vi "Washer HCC GUI.vi"(0 "Washer In":T1 {"Cycle Count" format="%05d"}, 2 "Enum":T5, 5 "Station Number In":string, 7 "New Washer Details In":T2, 9 "Com Port In":u8=13, 11 "Washer Status Serial Data In":T3, 12 "Agilent Data In":dbl[](array[numeric])=[1.0, 2.0, 3.0, 4.0, 5.0], 13 "Sample Buf Limit":i32=1000) -> (4 "Washer Out":T1 {"Cycle Count" format="%05d"}, 8 "New Dryer Testing File Init":bool, 10 "Restart Ready?":bool)   [LabVIEW 2009]
uses:
  Dryer Wilt/Update Wilt GUI Control.ctl
  Washer.ctl
  Dryer Wilt/Dryer Details.ctl
  Dryer Wilt/Dryer Com Port Info.ctl
  Dryer Wilt/Dryer Status Ctrl.ctl
  Globals HCC.vi
panel:
  out "Dryer Out.Sample Record(t, CC, Tc, ASCII, Status, L1,L2,Trmb,V{,V2,SW} ) 2":string[](array[string])
  out "Washer Out.Sample Record(t, CC, ASCII, Status )":string[](array[string])
  in  "Dryer Out":T1 {"Cycle Count" format="%05d"}
  in  "Tab Control":enum32{"Out", "In"}(tab)
  out "Washer Out  Breakout":T1 {"Cycle Count" format="%05d"}
  out "Washer In  Breakout":T6 {"Cycle Count" format="%05d"}
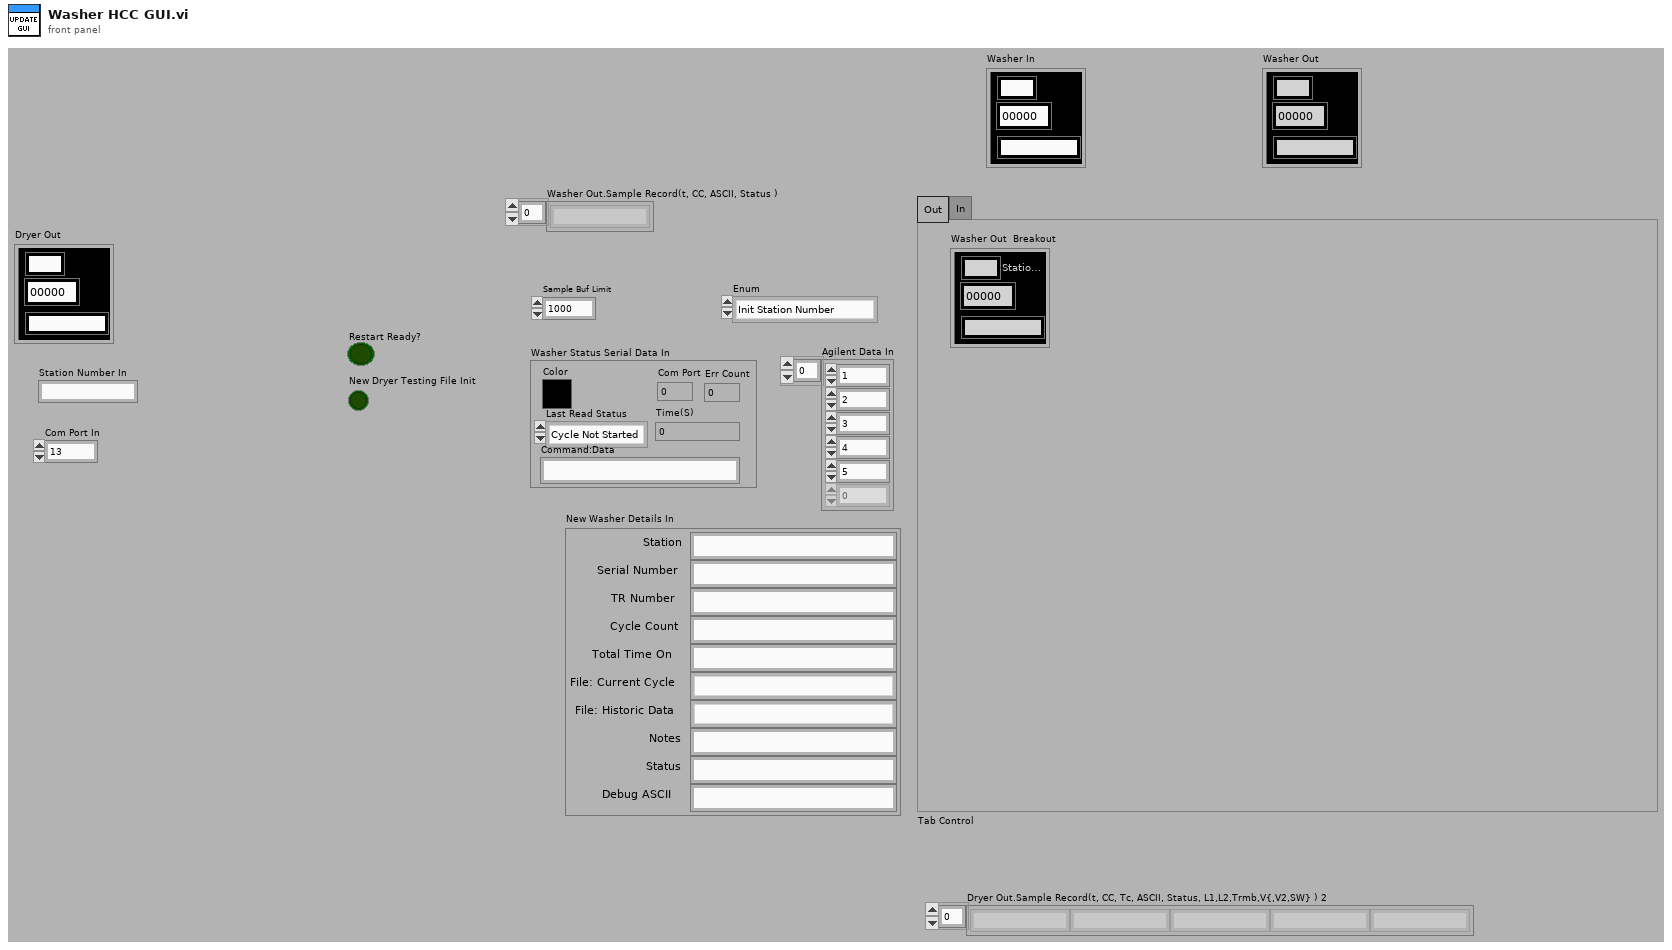
[diagram p1: front panel]
types:
  T1 = typedef "Washer.ctl" = cluster{"Serial Number":string, "Cycle Count":i32, "Station Number":string, "Dryer Details":T2, "Sample Record(t, CC, ASCII, Status ) ":string[], "Hist Record(Cycle Count, t-comp) ":string[][], "Status Color":u32, "Com Port":u8, "Bad Com Count":i32, "Boolean":bool}
  T2 = typedef "Dryer Details.ctl" = cluster{"Station":string, "Cycle Count":string, "Status":string, "Debug ASCII":string, "Notes":string, "File: Current Cycle":string, "Serial Number":string, "Total Time On":string, "TR Number":string, "File: Historic Data":string}
  T3 = typedef "Dryer Com Port Info.ctl" = cluster{"Color":u32, "Last Read Status":T4, "Command:Data":string, "Com Port":u8, "Time(S)":dbl, "Err Count":u8}
  T4 = typedef "Dryer Status Ctrl.ctl" = enum16{"Cycle Not Started", "Cycle Running", "Paused", "Cycle Completed", "Eval Mode Entered", "Err"}
  T5 = typedef "Update Wilt GUI Control.ctl" = enum16{"Init Station Number", "Update Detail Data", "Update Status", "Init Com Port Num", "Update Sample Info"}
  T6 = cluster{"Serial Number":string, "Cycle Count":i32, "Station Number":string, "Dryer Details":T2, "Sample Record(t, CC, Tc, ASCII, Status, L1,L2,Trmb,V{,V2,SW} ) ":string[], "Hist Record(Cycle Count, t-comp,L1max, L2max, Tmax) ":string[][], "Status Color":u32, "Com Port":u8, "Bad Com Count":i32, "Boolean":bool}
  T7 = cluster{"New Washer Details In":T2, "Station Number In":string, "Com Port In":u8, "Agilent Data In":dbl[], "Washer Status Serial Data In":T3, "Restart Ready?":bool, "Dryer Out":T1, "Sample Buf Limit":i32, "Temperature Fault":bool}
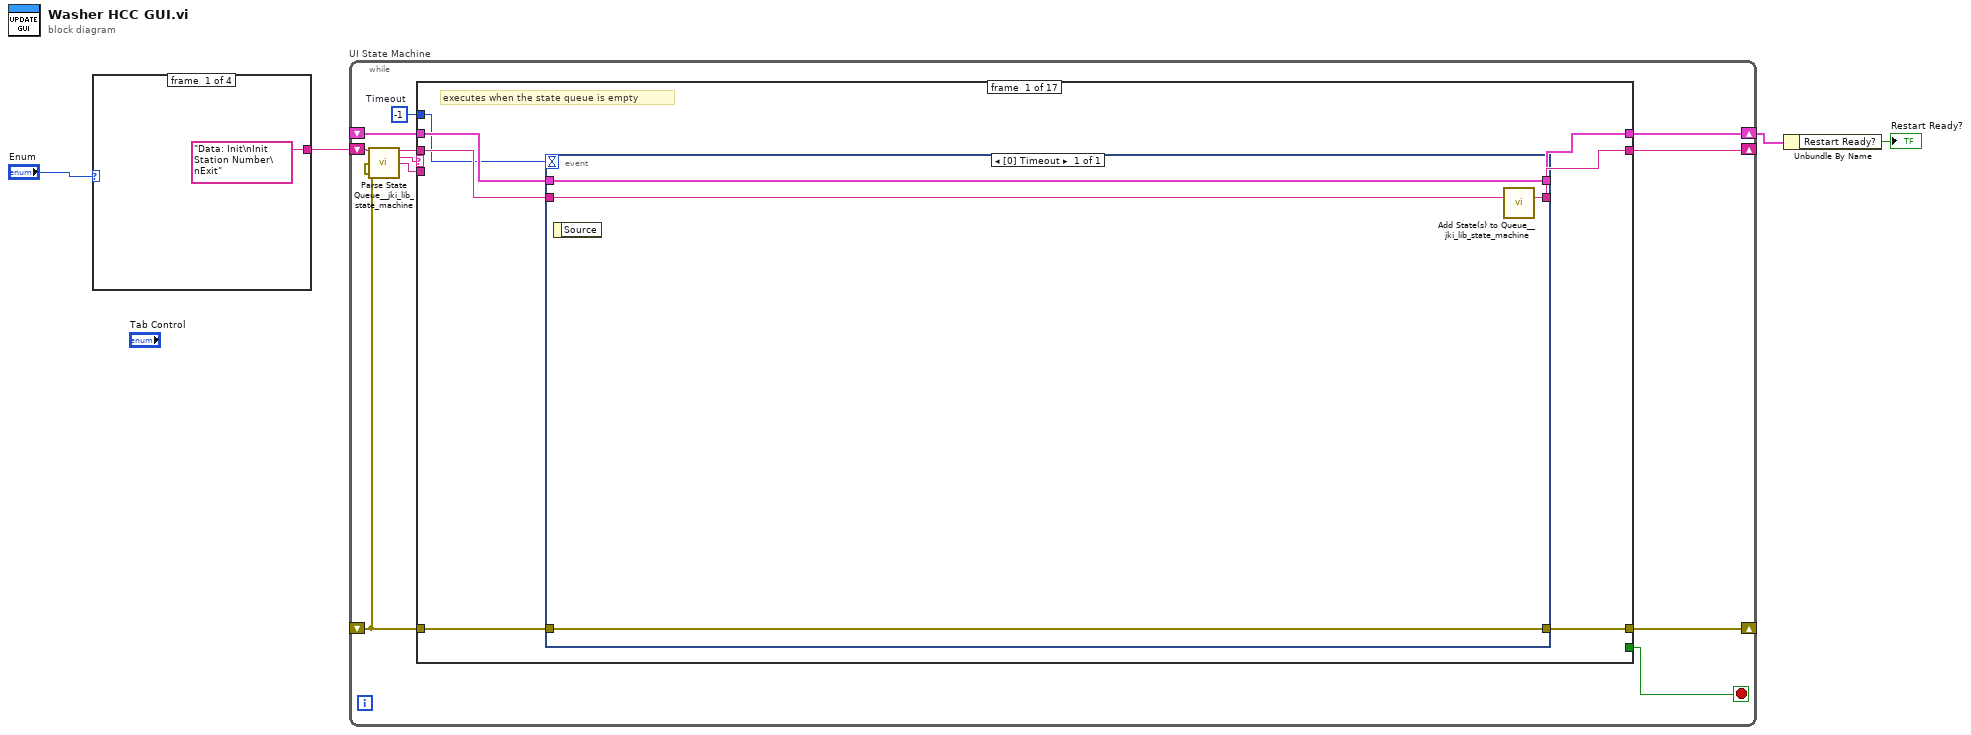
[diagram p0: block diagram]
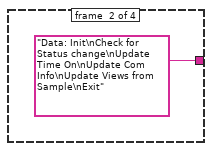
[diagram p2: hidden frame]
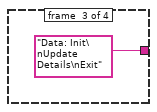
[diagram p3: hidden frame]
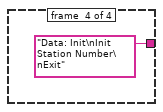
[diagram p4: hidden frame]
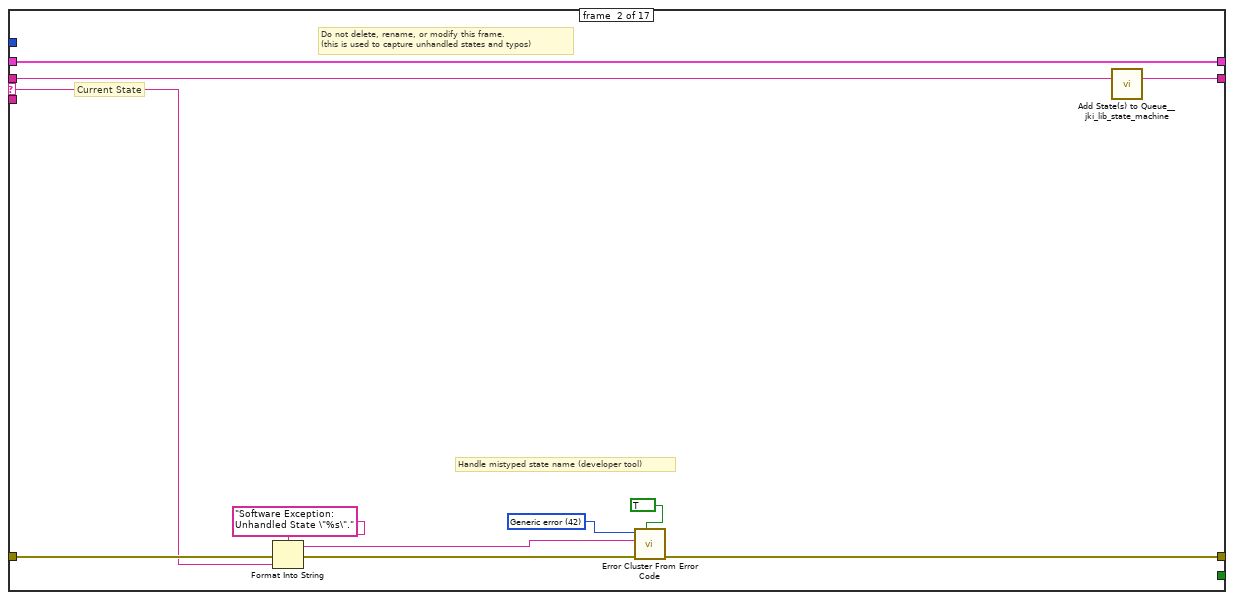
[diagram p5: hidden frame]
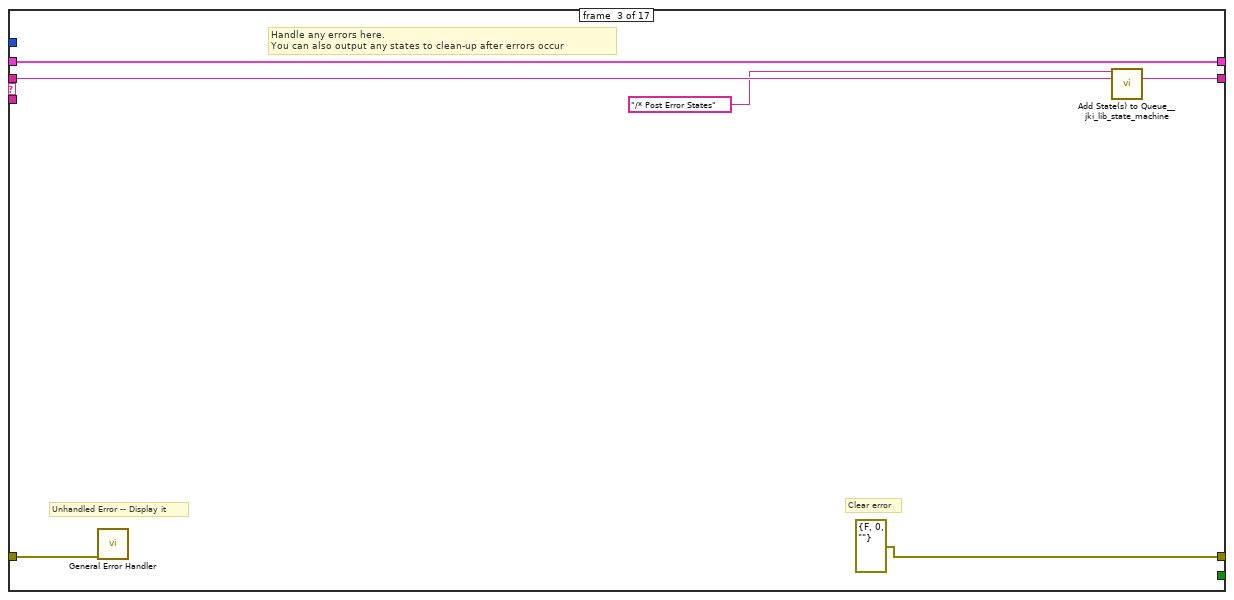
[diagram p6: hidden frame]
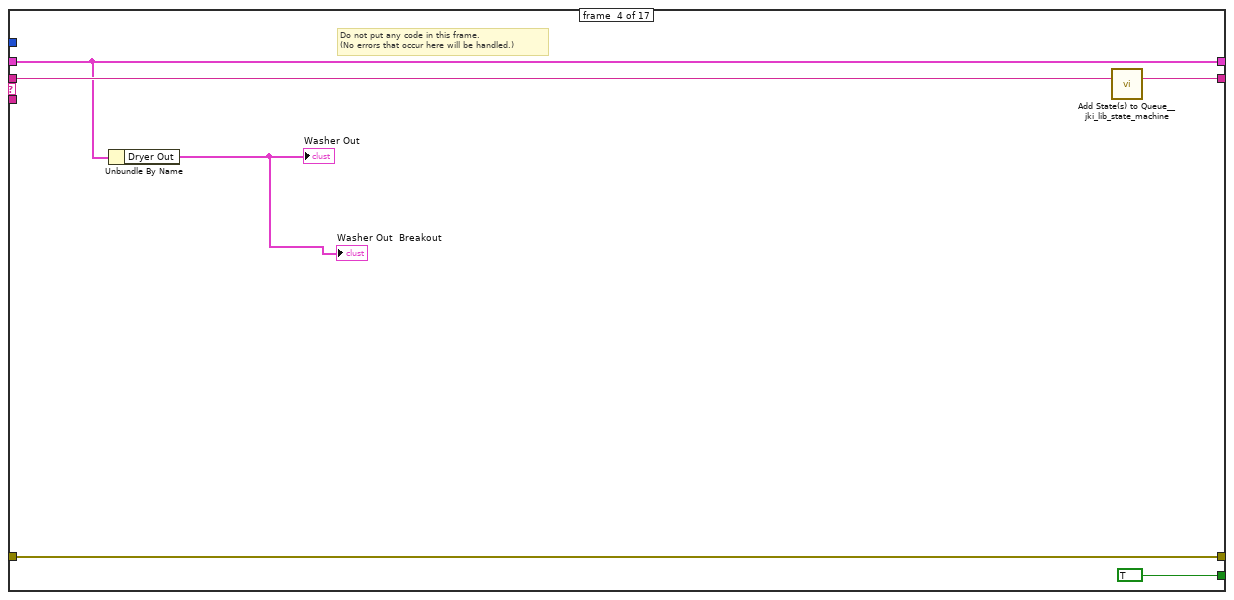
[diagram p7: hidden frame]
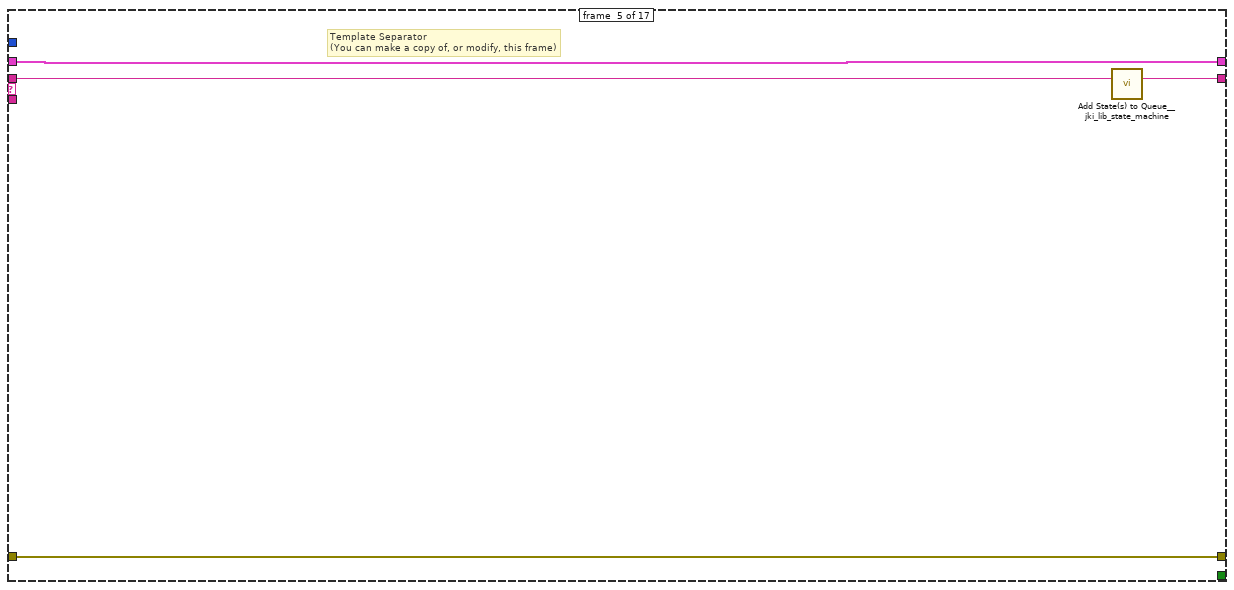
[diagram p8: hidden frame]
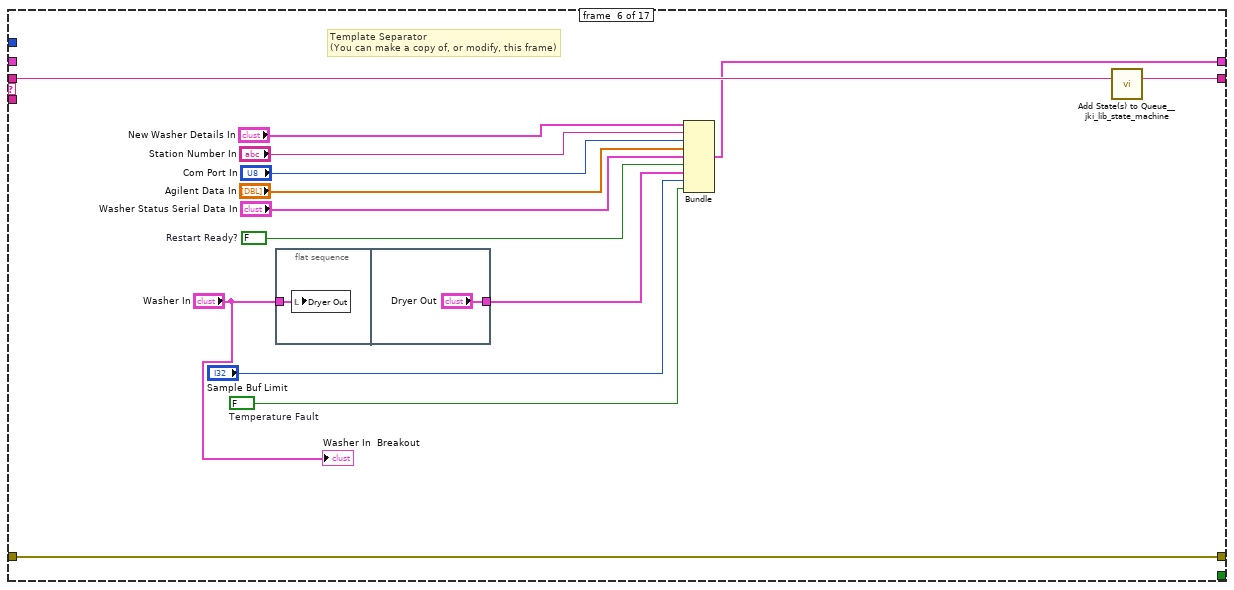
[diagram p9: hidden frame]
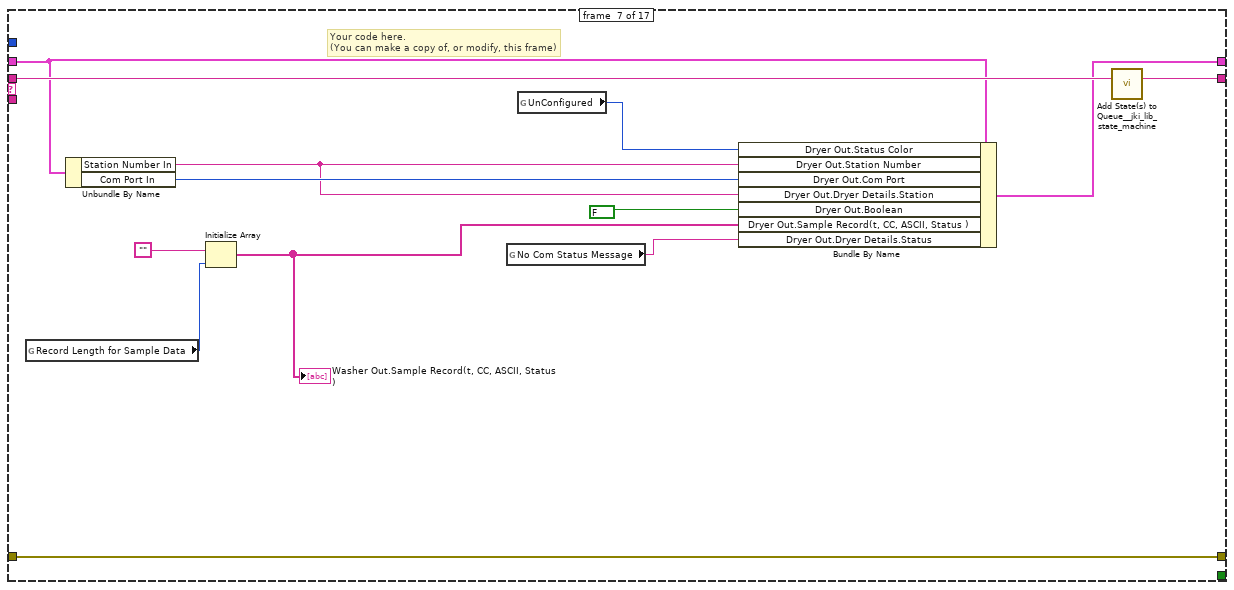
[diagram p10: hidden frame]
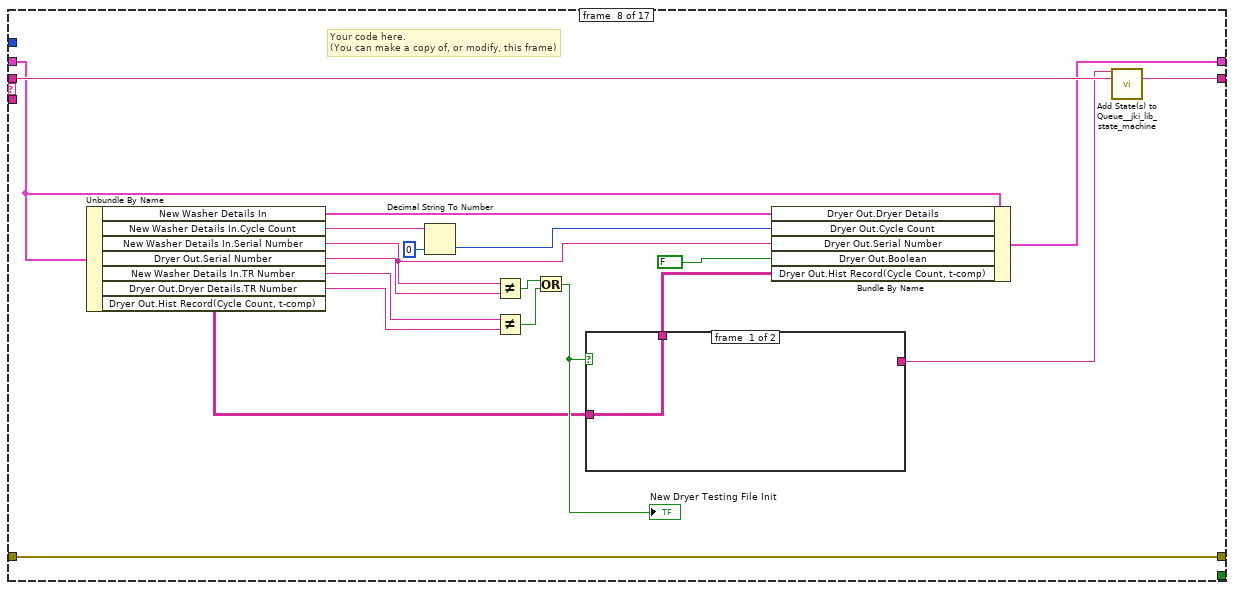
[diagram p11: hidden frame]
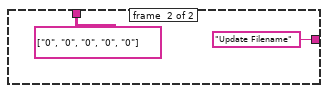
[diagram p12: hidden frame]
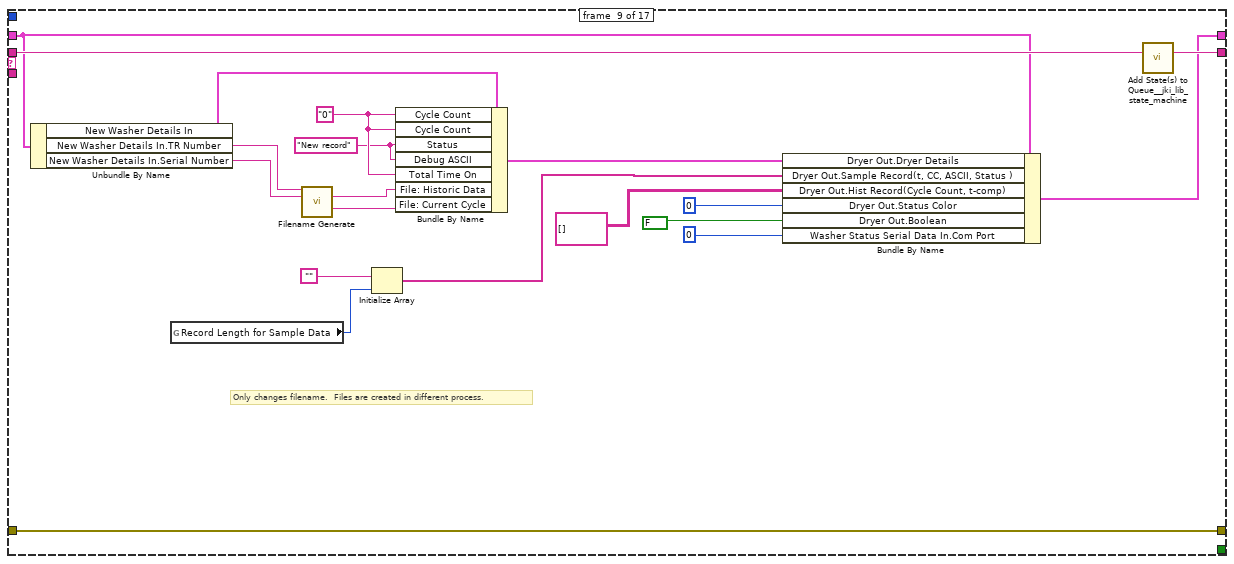
[diagram p13: hidden frame]
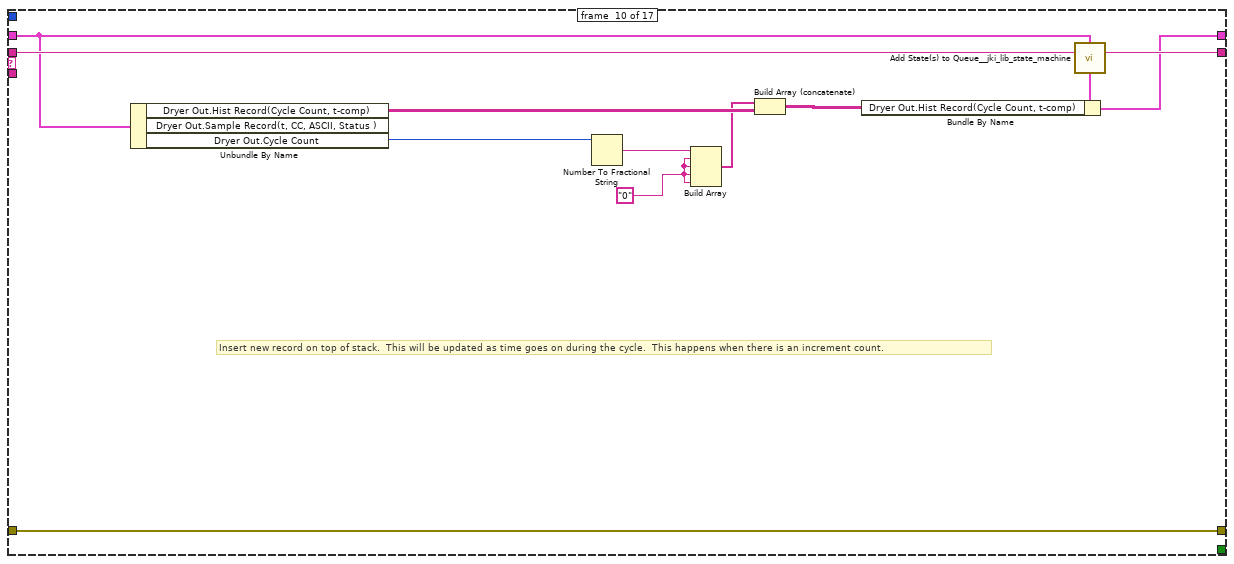
[diagram p14: hidden frame]
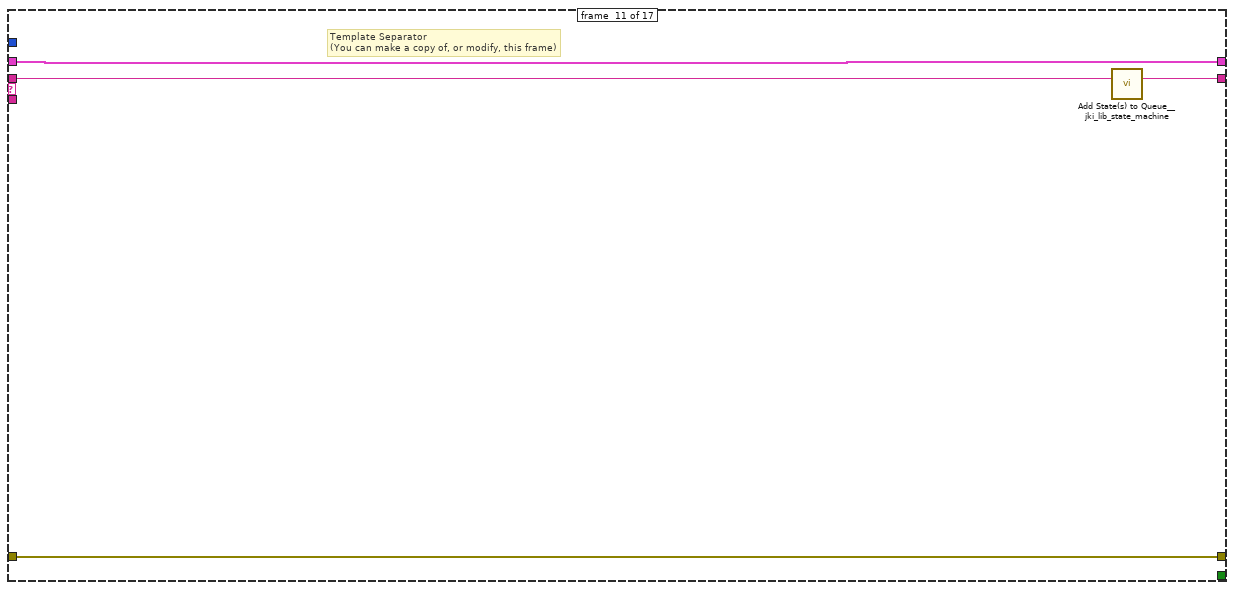
[diagram p15: hidden frame]
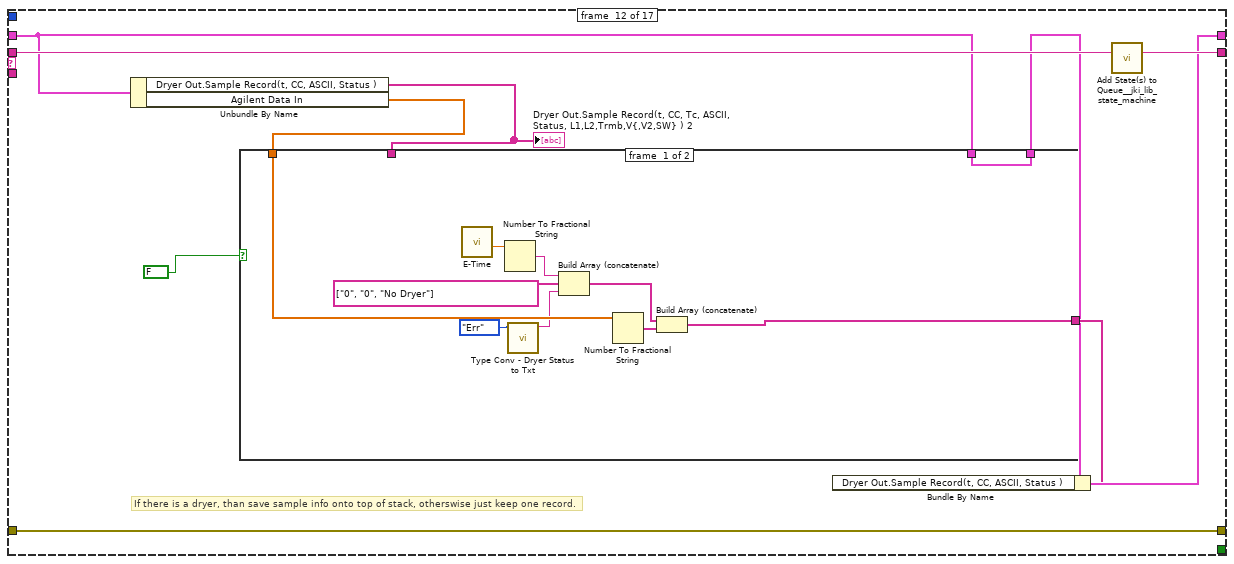
[diagram p16: hidden frame]
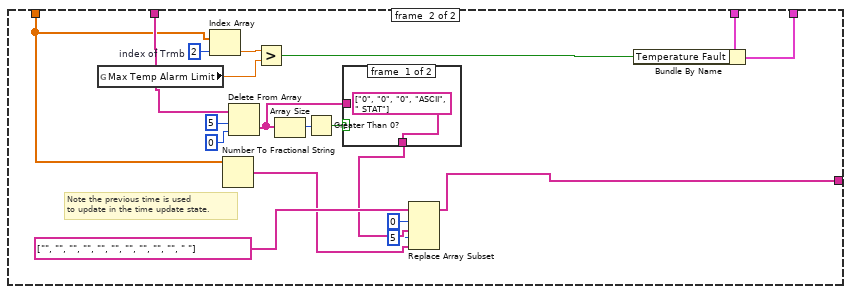
[diagram p17: hidden frame]
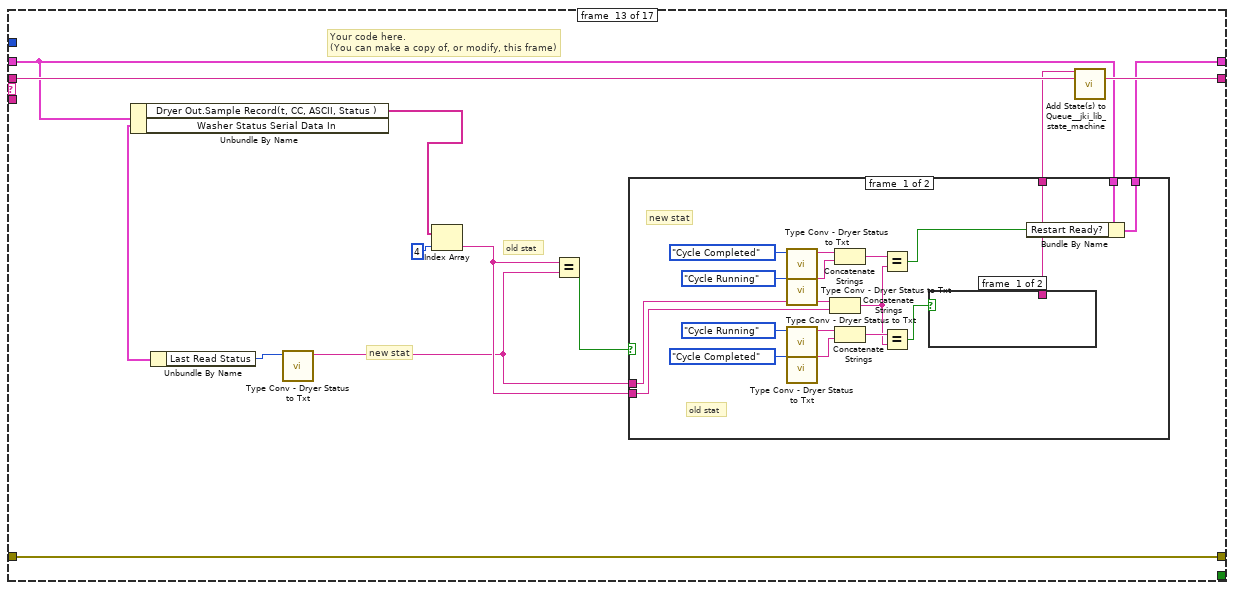
[diagram p19: hidden frame]
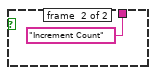
[diagram p20: hidden frame]
diagram:
  n1 = case shown="\"Update Detail Data\"" "Enum" {
    tunnel: ["Data: Init\nInit Station Number\nExit" ("States Out") "Data: Init\nCheck for Status change\nUpdate Time On\nUpdate Com Info\nUpdate Views from Sample\nExit" ("States Out") "Data: Init\nUpdate Details\nExit" ("States Out") "Data: Init\nInit Station Number\nExit" ("States Out")] -> w3
    frame #0 {
    }
    frame #1 {
    }
    frame #2 {
    }
    frame #3 {
    }
  }
  n2 = while "UI State Machine" {
    shift-right: [w12] -> w2
    shift-left: _ -> [w11]
    shift-right: [w15] -> _
    shift-left: _ -> [w9]
    shift-right: [w14] -> _
    shift-left: w3 -> [w16]
    stop <- w13 stop-if-true
    w10 = -1  # Timeout
    n3 = call <vilib>:"Parse State Queue__jki_lib_state_machine.vi"("State Queue"=w16, "Error In (no error)"=w9) -> ("Remaining States"=w18:string, "Current State"=w19:string, "Arguments"=w17:string)  [unwired: 11 in]
    n4 = case shown="\"Update Details\"" w19 {
      selector: w19 -> [_ w31 _ _ _ _ _ _ _ _ _ _ _ _ _ _ _]
      tunnel: w18 -> [w26 w35 w47 w53 w57 w71 w86 w106 w129 w140 w144 w154 w198 w229 w273 w329 w341]
      tunnel: w17 -> [_ _ _ _ _ _ _ _ _ _ _ _ _ _ _ _ _]
      tunnel: w11 -> [w24 w33 w44 w49 w54 _ w83 w97 w126 w137 w141 w146 w190 w222 w270 w326 w337]
      tunnel: [w23 w37 errorcluster {"status"=FALSE, "code"=0, "source"=""} ("error out") w51 w55 w69 w84 w104 w127 w138 w142 w152 w196 w227 w271 w327 w339] -> w15
      tunnel: w9 -> [w22 w36 w43 w51 w55 w69 w84 w104 w127 w138 w142 w152 w196 w227 w271 w327 w339]
      tunnel: [w25 w34 w46 w52 w56 w70 w85 w105 w128 w139 w143 w153 w197 w228 w272 w328 w340] -> w14
      tunnel: [_ _ _ TRUE _ _ _ _ _ _ _ _ _ _ _ _ _] -> w13
      tunnel: [w21 w33 w44 w49 w54 w68 w82 w103 w125 w136 w141 w151 w189 w221 w269 w325 w336] -> w12
      tunnel: w10 -> [w20 _ _ _ _ _ _ _ _ _ _ _ _ _ _ _ _]
      frame #0 {
        # "executes when the state queue is empty"
        n5 = event shown="[0] Timeout" {
          selector: _ -> [_]
          dyn-events: _ -> [_]
          timeout: w20 -> [_]
          tunnel: w26 -> [w30]
          tunnel: [w29] -> w25
          tunnel: w24 -> [w27]
          tunnel: [w28] -> w23
          tunnel: w22 -> [w28]
          tunnel: [w27] -> w21
          event [0] Timeout {
            n6 = event-data() -> ()  [unwired: 1 in, 1 out]
            n7 = call <vilib>:"Add State(s) to Queue__jki_lib_state_machine.vi"("State(s) in (\"\")"=w30) -> ("States Out"=w29:string)  [unwired: 14 in]
          }
        }
      }
      frame #1 {
        w40 = 42 items=["No error", "Argument error", "Memory is full", "Out of zone", "End of file", "File already open", "Generic file I/O error", "File not found", "File permission error", "Disk is full", "Duplicate path", "Too many files open", "System feature not enabled", "Resource file not found", "Cannot add resource", "Resource not found", "Image not found", "Image memory error", "Pen does not exist", "Config type invalid", "Config token not found", "Config parse error", "Config memory error", "Bad external code format", "Bad external code offset", "External code not present", "Null window", "Destroy window error", "Null menu", "Print aborted", "Bad print record", "Print driver error", "Windows error during printing", "Memory error during printing", "Print dialog error", "Generic print error", "Invalid device refnum", "Device not found", "Device parameter error", "Device unit error", "Cannot open device", "Device call aborted", "Generic error", "Cancelled by user", "Object ID too low", "Object ID too high", "Object not in heap", "Unknown heap", "Unknown object (invalid DefProc)", "Unknown object (DefProc not in table)", "Message out of range", "Invalid (null) method", "Unknown message", "Manager call not supported", "Bad address", "Network operation in progress", "Network operation timed out", "Connection is busy", "Network attribute not supported", "Network error", "Address in use", "System out of memory", "Connection aborted", "Connection refused", "Not connected", "Already connected", "Connection closed", "Initialization error (interapplication manager)", "Bad occurrence", "Wait on unbound occurrence handler", "Occurrence queue overflow", "Datalog type conflict", "Unused", "Unrecognized type (interapplication manager)", "Memory corrupt", "Failed to make temporary DLL", "Old CIN version", "Drag socket not found", "Failed to load drop-object", "Failed to register OLE object", "Failed to release OLE object", "Format specifier type mismatch", "Unknown format specifier", "Too few format specifiers", "Too many format specifiers", "Scan failed", "Newer CIN version", "Error converting to variant", "Runtime menu error", "Password tampered", "Variant attribute not found", "Incompatible variant data type", "Event data is not available", "Event Store is not present", "Occurrence is not found", "Event Queue is not created", "Event info is not available", "Refnum passed is NULL", "Error retrieving Class GUID", "Error retrieving CoClass GUID", "Error retrieving TypeLib GUID.", "Bad built application magic bytes.", "Specific driver is different from the specific driver associated with the Logical Name.", "There is no session opened to the class driver.", "Max Error", "MAX - Error with config objects", "MAX - Error loading configuration", "MAX - Group not supported"]
        # "Current State"
        # "Do not delete, rename, or modify this frame.\n(this is used to capture unhandled states and typos)"
        # "Handle mistyped state name (developer tool)"
        n8 = Format Into String(format string="Software Exception: Unhandled State \"%s\"." ("message"), error in=w36, w31) -> (resulting string=w39:string, error out=w38:errorcluster)  [unwired: 1 in]
        n9 = call <vilib>:"Error Cluster From Error Code.vi"("show call chain? (False)"=TRUE, "error in (no error)"=w38, "error message (\"\")"=w39, "error code (0)"=w40) -> ("error out"=w37:errorcluster)  [unwired: 5 in]
        n10 = call <vilib>:"Add State(s) to Queue__jki_lib_state_machine.vi"("State(s) in (\"\")"=w35) -> ("States Out"=w34:string)  [unwired: 14 in]
      }
      frame #2 {
        # "Unhandled Error -- Display it"
        # "Handle any errors here.\nYou can also output any states to clean-up after errors occur"
        # "Clear error"
        n11 = call <vilib>:"General Error Handler.vi"("error in (no error)"=w43) -> ()  [unwired: 10 in, 5 out]
        n12 = call <vilib>:"Add State(s) to Queue__jki_lib_state_machine.vi"("State(s) in Front (\"\")"="/* Post Error States", "State(s) in (\"\")"=w47) -> ("States Out"=w46:string)  [unwired: 13 in]
      }
      frame #3 {
        # "Do not put any code in this frame.\n(No errors that occur here will be handled.)"
        n13 = Unbundle By Name(w49) -> ("Dryer Out"=→"Washer Out" →"Washer Out  Breakout":T1)
        n14 = call <vilib>:"Add State(s) to Queue__jki_lib_state_machine.vi"("State(s) in (\"\")"=w53) -> ("States Out"=w52:string)  [unwired: 14 in]
      }
      frame #4 {
        # "Template Separator\n(You can make a copy of, or modify, this frame)"
        n15 = call <vilib>:"Add State(s) to Queue__jki_lib_state_machine.vi"("State(s) in (\"\")"=w57) -> ("States Out"=w56:string)  [unwired: 14 in]
      }
      frame #5 {
        w58 = FALSE  # Temperature Fault
        w62 = FALSE  # Restart Ready?
        # "Template Separator\n(You can make a copy of, or modify, this frame)"
        n16 = flat-sequence {
          tunnel: "Washer In" -> [w72]
          tunnel: ["Dryer Out"] -> w60
          frame #0 {
            n17 = local write "Dryer Out"(w72) -> ()
          }
          frame #1 {
          }
        }
        n18 = Bundle("New Washer Details In"="New Washer Details In", "Station Number In"="Station Number In", "Com Port In"="Com Port In", "Agilent Data In"="Agilent Data In", "Washer Status Serial Data In"="Washer Status Serial Data In", "Restart Ready?"=w62, "Dryer Out"=w60, "Sample Buf Limit"="Sample Buf Limit", "Temperature Fault"=w58) -> (w68:T7)  [unwired: 1 in]
        n19 = call <vilib>:"Add State(s) to Queue__jki_lib_state_machine.vi"("State(s) in (\"\")"=w71) -> ("States Out"=w70:string)  [unwired: 14 in]
        "Washer In  Breakout" <- "Washer In"
      }
      frame #6 {
        # "Your code here.\n(You can make a copy of, or modify, this frame)"
        n20 = global read "Globals HCC.vi" "Record Length for Sample Data"() -> (w75:i32)
        n21 = Unbundle By Name(w83) -> ("Station Number In"=w74:string, "Com Port In"=w81:u8)
        n22 = Initialize Array("", w75) -> (w76:string[])
        "Washer Out.Sample Record(t, CC, ASCII, Status )" <- w76
        n23 = global read "Globals HCC.vi" "No Com Status Message"() -> (w78:string)
        n24 = global read "Globals HCC.vi" "UnConfigured"() -> (w79:u32)
        n25 = Bundle By Name(cluster=w83, "Dryer Out.Status Color"=w79, "Dryer Out.Station Number"=w74, "Dryer Out.Com Port"=w81, "Dryer Out.Dryer Details.Station"=w74, "Dryer Out.Boolean"=FALSE ("Dryer In.Boolean"), "Dryer Out.Sample Record(t, CC, ASCII, Status )"=w76, "Dryer Out.Dryer Details.Status"=w78) -> (w82:T7)
        n26 = call <vilib>:"Add State(s) to Queue__jki_lib_state_machine.vi"("State(s) in (\"\")"=w86) -> ("States Out"=w85:string)  [unwired: 14 in]
      }
      frame #7 {
        # "Your code here.\n(You can make a copy of, or modify, this frame)"
        n27 = Unbundle By Name(w97) -> ("New Washer Details In"=w96:T2, "New Washer Details In.Cycle Count"=w93:string, "New Washer Details In.Serial Number"=w92:string, "Dryer Out.Serial Number"=w91:string, "New Washer Details In.TR Number"=w95:string, "Dryer Out.Dryer Details.TR Number"=w94:string, "Dryer Out.Hist Record(Cycle Count, t-comp)"=w87:string[][])
        n28 = Decimal String To Number(string=w93, default (0L)=0 ("default (0 I32)")) -> (number=w100:i32)  [unwired: 1 in, 1 out]
        n29 = Not Equal?(x=w92, y=w91) -> (x != y?=w90:bool)
        n30 = Not Equal?(x=w95, y=w94) -> (x != y?=w89:bool)
        n31 = Or(x=w90, y=w89) -> (x .or. y?=w101:bool)
        "New Dryer Testing File Init" <- w101
        n32 = case shown="False" w101 {
          tunnel: [_ "Update Filename"] -> w102
          tunnel: [w107 string[][] [["0", "0", "0", "0", "0"]] ("Hist Record(Cycle Count, t-comp,L1max, L2max, Tmax)")] -> w88
          tunnel: w87 -> [w107 _]
          frame #0 {
          }
          frame #1 {
          }
        }
        n33 = Bundle By Name(cluster=w97, "Dryer Out.Dryer Details"=w96, "Dryer Out.Cycle Count"=w100, "Dryer Out.Serial Number"=w92, "Dryer Out.Boolean"=FALSE ("Dryer In.Boolean"), "Dryer Out.Hist Record(Cycle Count, t-comp)"=w88) -> (w103:T7)
        n34 = call <vilib>:"Add State(s) to Queue__jki_lib_state_machine.vi"("State(s) in Front (\"\")"=w102, "State(s) in (\"\")"=w106) -> ("States Out"=w105:string)  [unwired: 13 in]
      }
      frame #8 {
        w123 = "New record" ("Status")
        w124 = "0" ("Cycle Count")
        # "Only changes filename.  Files are created in different process."
        n35 = Unbundle By Name(w126) -> ("New Washer Details In"=w121:T2, "New Washer Details In.TR Number"=w119:string, "New Washer Details In.Serial Number"=w118:string)
        n36 = global read "Globals HCC.vi" "Record Length for Sample Data"() -> (w110:i32)
        n37 = call "Filename Generate.vi"("TR Number"=w119, "Serial Number"=w118) -> ("Filename for Hist data"=w120:string, "Filename for Samples"=w113:string)  [unwired: 10 in, 2 out]
        n38 = Initialize Array("", w110) -> (w111:string[])
        n39 = Bundle By Name(cluster=w121, "Cycle Count"=w124, "Cycle Count"=w124, "Status"=w123, "Debug ASCII"=w123, "Total Time On"=w124, "File: Historic Data"=w120, "File: Current Cycle"=w113) -> (w122:T2)
        n40 = Bundle By Name(cluster=w126, "Dryer Out.Dryer Details"=w122, "Dryer Out.Sample Record(t, CC, ASCII, Status )"=w111, "Dryer Out.Hist Record(Cycle Count, t-comp)"=string[][] [] ("Dryer In.Sample Record(t, CC, Tc, ASCII, Status, L1,L2,Trmb,V{,V2,SW} )"), "Dryer Out.Status Color"=u32 0 ("Dryer In.Status Color"), "Dryer Out.Boolean"=FALSE ("Dryer In.Boolean"), "Washer Status Serial Data In.Com Port"=u8 0 ("Dryer In.Com Port")) -> (w125:T7)
        n41 = call <vilib>:"Add State(s) to Queue__jki_lib_state_machine.vi"("State(s) in (\"\")"=w129) -> ("States Out"=w128:string)  [unwired: 14 in]
      }
      frame #9 {
        w130 = "0" ("element")
        # "Insert new record on top of stack.  This will be updated as time goes on during the cycle.  This happens when there is an increment count."
        n42 = Unbundle By Name(w137) -> ("Dryer Out.Hist Record(Cycle Count, t-comp)"=w134:string[][], "Dryer Out.Cycle Count"=w131:i32)  [unwired: 1 out]
        n43 = Number To Fractional String(number=w131) -> (F-format string=w135:string)  [unwired: 3 in]
        n44 = Build Array(w135, w130, w130, w130, w130) -> (w133:string[])
        n45 = Build Array (concatenate)(w133, w134) -> (w132:string[][])
        n46 = Bundle By Name(cluster=w137, "Dryer Out.Hist Record(Cycle Count, t-comp)"=w132) -> (w136:T7)
        n47 = call <vilib>:"Add State(s) to Queue__jki_lib_state_machine.vi"("State(s) in (\"\")"=w140) -> ("States Out"=w139:string)  [unwired: 14 in]
      }
      frame #10 {
        # "Template Separator\n(You can make a copy of, or modify, this frame)"
        n48 = call <vilib>:"Add State(s) to Queue__jki_lib_state_machine.vi"("State(s) in (\"\")"=w144) -> ("States Out"=w143:string)  [unwired: 14 in]
      }
      frame #11 {
        # "If there is a dryer, than save sample info onto top of stack, otherswise just keep one record."
        n49 = Unbundle By Name(w146) -> ("Dryer Out.Sample Record(t, CC, ASCII, Status )"=w148:string[], "Agilent Data In"=w150:dbl[])
        "Dryer Out.Sample Record(t, CC, Tc, ASCII, Status, L1,L2,Trmb,V{,V2,SW} ) 2" <- w148
        n50 = case shown="False" FALSE {
          tunnel: w150 -> [w164 w171]
          tunnel: [w156 w172] -> w149
          tunnel: w148 -> [_ w173]
          tunnel: w146 -> [w155 w167]
          tunnel: [w155 w166] -> w145
          frame #0 {
            n51 = call "E-Time.vi"() -> ("Elapsed Time (sec)"=w158:dbl)  [unwired: 9 in, 2 out]
            n52 = Number To Fractional String(number=w158) -> (F-format string=w157:string)  [unwired: 3 in]
            n53 = call "Type Conv - Dryer Status to Txt.vi"("Status"=Dryer_Status_Ctrl."Err") -> ("Ring Text.Text"=w160:string)  [unwired: 10 in]
            n54 = Build Array (concatenate)(w157, string[] ["0", "0", "No Dryer"], w160) -> (w159:string[])
            n55 = Number To Fractional String(number=w164) -> (F-format string=w163:string[])  [unwired: 3 in]
            n56 = Build Array (concatenate)(w159, w163) -> (w156:string[])
          }
          frame #1 {
            w170 = 2  # index of Trmb
            # "Note the previous time is used\nto update in the time update state."
            n57 = global read "Globals HCC.vi" "Max Temp Alarm Limit"() -> (w168:dbl)
            n58 = Index Array(array=w171, index=w170) -> (element=w169:dbl)
            n59 = Number To Fractional String(number=w171) -> (F-format string=w174:string[])  [unwired: 3 in]
            n60 = Delete From Array(array=w173, length=5, index=0) -> (deleted portion=w179:string[])  [unwired: 1 out]
            n61 = Greater?(x=w169, y=w168) -> (0:w165:bool)
            n62 = Array Size(array=w179) -> (size(s)=w181:i32)
            n63 = Greater Than 0?(x=w181) -> (x > 0?=w180:bool)
            n64 = case shown="True" w180 {
              tunnel: [string[] ["0", "0", "0", "ASCII", " STAT"] w185] -> w176
              tunnel: w179 -> [_ w185]
              frame #0 {
              }
              frame #1 {
              }
            }
            n65 = Replace Array Subset(array=string[] ["", "", "", "", "", "", "", "", "", "", " "], new element #1=w176, index #1=0 ("index"), new element #2=w174, index #2=5 ("index")) -> (w172:string[])
            n66 = Bundle By Name(cluster=w167, "Temperature Fault"=w165) -> (w166:T7)
          }
        }
        n67 = Bundle By Name(cluster=w145, "Dryer Out.Sample Record(t, CC, ASCII, Status )"=w149) -> (w151:T7)
        n68 = call <vilib>:"Add State(s) to Queue__jki_lib_state_machine.vi"("State(s) in (\"\")"=w154) -> ("States Out"=w153:string)  [unwired: 14 in]
      }
      frame #12 {
        # "new stat"
        # "old stat"
        # "Your code here.\n(You can make a copy of, or modify, this frame)"
        n69 = Unbundle By Name(w190) -> ("Dryer Out.Sample Record(t, CC, ASCII, Status )"=w194:string[], "Washer Status Serial Data In"=w195:T3)
        n70 = Unbundle By Name(w195) -> ("Last Read Status"=w193:T4)
        n71 = call "Type Conv - Dryer Status to Txt.vi"("Status"=w193) -> ("Ring Text.Text"=w187:string)  [unwired: 10 in]
        n72 = Index Array(array=w194, index=4 ("disabled index (col)")) -> (element=w188:string)
        n73 = Equal?(x=w188, y=w187) -> (x = y?=w192:bool)
        n74 = case shown="False" w192 {
          tunnel: [w205 "" ("State(s) in Front (\"\")")] -> w191
          tunnel: w187 -> [w212 _]
          tunnel: w188 -> [w211 _]
          tunnel: w190 -> [w201 w218]
          tunnel: [w200 w218] -> w189
          frame #0 {
            # "new stat"
            # "old stat"
            n75 = call "Type Conv - Dryer Status to Txt.vi"("Status"=Dryer_Status_Ctrl."Cycle Completed") -> ("Ring Text.Text"=w209:string)  [unwired: 10 in]
            n76 = call "Type Conv - Dryer Status to Txt.vi"("Status"=Dryer_Status_Ctrl."Cycle Running") -> ("Ring Text.Text"=w210:string)  [unwired: 10 in]
            n77 = call "Type Conv - Dryer Status to Txt.vi"("Status"=Dryer_Status_Ctrl."Cycle Running") -> ("Ring Text.Text"=w214:string)  [unwired: 10 in]
            n78 = call "Type Conv - Dryer Status to Txt.vi"("Status"=Dryer_Status_Ctrl."Cycle Completed") -> ("Ring Text.Text"=w213:string)  [unwired: 10 in]
            n79 = Concatenate Strings(w212, w211) -> (w203:string)
            n80 = Concatenate Strings(w209, w210) -> (w206:string)
            n81 = Concatenate Strings(w214, w213) -> (w204:string)
            n82 = Equal?(x=w206, y=w203) -> (x = y?=w199:bool)
            n83 = Equal?(x=w204, y=w203) -> (x = y?=w202:bool)
            n84 = case shown="True" w202 {
              tunnel: [_ "Increment Count" ("State(s) in Front (\"\")")] -> w205
              frame #0 {
              }
              frame #1 {
              }
            }
            n85 = Bundle By Name(cluster=w201, "Restart Ready?"=w199) -> (w200:T7)
          }
          frame #1 {
            # "If status is the same,\ndon't do extra steps."
          }
        }
        n86 = call <vilib>:"Add State(s) to Queue__jki_lib_state_machine.vi"("State(s) in Front (\"\")"=w191, "State(s) in (\"\")"=w198) -> ("States Out"=w197:string)  [unwired: 13 in]
      }
      frame #13 {
        # "Your code here.\n(You can make a copy of, or modify, this frame)"
        n87 = Unbundle By Name(w222) -> ("Dryer Out.Sample Record(t, CC, ASCII, Status )"=w224:string[], "Washer Status Serial Data In.Time(S)"=w223:dbl, "Washer Status Serial Data In.Last Read Status"=w226:T4)
        n88 = Equal?(x=w226, y=Dryer_Status_Ctrl."Cycle Running" ("Status")) -> (x = y?=w225:bool)
        n89 = case shown="True" w225 {
          tunnel: w224 -> [w238 w251]
          tunnel: w223 -> [w234 w249]
          tunnel: w222 -> [w240 w253]
          tunnel: [w239 w252] -> w221
          frame #0 {
            # "Cum Time"
            # "Current Rec Time"
            # "Last Time"
            n90 = Index Array(array=w238, index #1=0 ("index (row)"), index #2=2 ("disabled index (col)")) -> (element #1=w246:string, element #2=w242:string)
            n91 = Fract/Exp String To Number(string=w246) -> (number=w243:dbl)  [unwired: 3 in, 1 out]
            n92 = Fract/Exp String To Number(string=w242) -> (number=w241:dbl)  [unwired: 3 in, 1 out]
            n93 = Subtract(x=w234, y=w243) -> (x-y=w244:dbl)
            n94 = Add(x=w244, y=w241) -> (x+y=w236:dbl)
            n95 = Number To Fractional String(number=w234) -> (F-format string=w233:string)  [unwired: 3 in]
            n96 = Number To Fractional String(number=w236) -> (F-format string=w235:string)  [unwired: 3 in]
            n97 = Replace Array Subset(array=w238, new element #1=w235, index #1=2 ("index (row)"), new element #2=w233, index #2=0 ("index")) -> (w237:string[])
            n98 = Bundle By Name(cluster=w240, "Dryer Out.Sample Record(t, CC, ASCII, Status )"=w237) -> (w239:T7)
          }
          frame #1 {
            # "Just update Record Time"
            n99 = Number To Fractional String(number=w249) -> (F-format string=w247:string)  [unwired: 3 in]
            n100 = Replace Array Subset(array=w251, new element=w247, index=0 ("index (row)")) -> (w250:string[])
            n101 = Bundle By Name(cluster=w253, "Dryer Out.Sample Record(t, CC, ASCII, Status )"=w250) -> (w252:T7)
          }
        }
        n102 = call <vilib>:"Add State(s) to Queue__jki_lib_state_machine.vi"("State(s) in (\"\")"=w229) -> ("States Out"=w228:string)  [unwired: 14 in]
      }
      frame #14 {
        # "Your code here.\n(You can make a copy of, or modify, this frame)"
        n103 = Unbundle By Name(w270) -> ("Temperature Fault"=w256:bool, "Dryer Out.Sample Record(t, CC, ASCII, Status )"=w268:string[], "Washer Status Serial Data In"=w267:T3)
        n104 = Unbundle By Name(w267) -> ("Err Count"=w263:u8, "Color"=w257:u32, "Last Read Status"=w264:T4, "Command:Data"=w259:string)
        n105 = disable-structure shown="Enabled" {
          disable-tunnel: w259 -> [w279 w280]
          disable-tunnel: [w274 w280] -> w258
          frame #0 {
            w275 = " :: " ("replace string (\"\")")
            n106 = Search and Replace String(input string=w279, search string="\r\n", replace string=w275) -> (result string=w277:string)  [unwired: 5 in, 3 out]
            n107 = Search and Replace String(input string=w277, search string="\r", replace string=w275) -> (result string=w274:string)  [unwired: 5 in, 3 out]
          }
          frame #1 {
          }
        }
        n108 = global read "Globals HCC.vi" "Fault Color"() -> (w255:u32)
        n109 = call "Type Conv - Dryer Status to Txt.vi"("Status"=w264) -> ("Ring Text.Text"=w266:string)  [unwired: 10 in]
        n110 = Select(t=w255, s=w256, f=w257) -> (s? t:f=w254:u32)
        n111 = To Long Integer(number=w263) -> (32bit integer=w262:i32)
        n112 = Replace Array Subset(array=w268, new element #1=w258, index #1=3 ("disabled index (col)"), new element #2=w266, index #2=4 ("disabled index (col)")) -> (w265:string[])
        n113 = Bundle By Name(cluster=w270, "Dryer Out.Bad Com Count"=w262, "Dryer Out.Status Color"=w254, "Dryer Out.Sample Record(t, CC, ASCII, Status )"=w265) -> (w269:T7)
        n114 = call <vilib>:"Add State(s) to Queue__jki_lib_state_machine.vi"("State(s) in (\"\")"=w273) -> ("States Out"=w272:string)  [unwired: 14 in]
      }
      frame #15 {
        w285 = 4  # Tmax
        w309 = 3  # L2max
        w310 = 2  # L1max
        w311 = 1  # t-comp
        w313 = 0 ("index (row)")
        w312 = 0  # CC
        w287 = 0 ("index (row)")
        w319 = 1  # CC(col)
        # "Updates the view data, and the History data."
        # "Your code here.\n(You can make a copy of, or modify, this frame)"
        n115 = Unbundle By Name(w326) -> ("Dryer Out.Sample Record(t, CC, ASCII, Status )"=w324:string[], "Dryer Out.Hist Record(Cycle Count, t-comp)"=w315:string[][])
        n116 = Index Array(array=w315, index (row) #1=w287, index (col) #1=2 ("disabled index (col)"), index (row) #2=w287, index (col) #2=3 ("disabled index (col)"), index (row) #3=w287, index (col) #3=4 ("disabled index (col)")) -> (element #1=w297:string, element #2=w296:string, element #3=w282:string)
        n117 = Index Array(array=w324, index #1=w319, index #2=4 ("disabled index (col)"), index #3=3 ("disabled index (col)"), index #4=2 ("disabled index (col)"), index #5=5 ("disabled index (col)"), index #6=6 ("disabled index (col)"), index #7=7 ("disabled index (col)")) -> (element #1=w308:string, element #2=w322:string, element #3=w321:string, element #4=w307:string, element #5=w298:string, element #6=w295:string, element #7=w283:string)
        n118 = Fract/Exp String To Number(string=w298) -> (number=w302:dbl)  [unwired: 3 in, 1 out]
        n119 = Fract/Exp String To Number(string=w297) -> (number=w301:dbl)  [unwired: 3 in, 1 out]
        n120 = Fract/Exp String To Number(string=w295) -> (number=w303:dbl)  [unwired: 3 in, 1 out]
        n121 = Fract/Exp String To Number(string=w296) -> (number=w304:dbl)  [unwired: 3 in, 1 out]
        n122 = Fract/Exp String To Number(string=w283) -> (number=w289:dbl)  [unwired: 3 in, 1 out]
        n123 = Fract/Exp String To Number(string=w282) -> (number=w288:dbl)  [unwired: 3 in, 1 out]
        n124 = Max & Min(x=w302, y=w301) -> (max(x,y)=w291:dbl)  [unwired: 1 out]
        n125 = Max & Min(x=w303, y=w304) -> (max(x,y)=w292:dbl)  [unwired: 1 out]
        n126 = Max & Min(x=w289, y=w288) -> (max(x,y)=w290:dbl)  [unwired: 1 out]
        n127 = Number To Fractional String(number=w291) -> (F-format string=w294:string)  [unwired: 3 in]
        n128 = Number To Fractional String(number=w292) -> (F-format string=w293:string)  [unwired: 3 in]
        n129 = Number To Fractional String(number=w290) -> (F-format string=w286:string)  [unwired: 3 in]
        n130 = Fract/Exp String To Number(string=w308, default (0 dbl)=0 ("default (0 DBL)")) -> (number=w323:i32)  [unwired: 2 in, 1 out]
        n131 = Replace Array Subset(array=w315, new element #1=w308, index (row) #1=w313, index (col) #1=w312, new element #2=w307, index (row) #2=w313, index (col) #2=w311, new element #3=w294, index (row) #3=w313, index (col) #3=w310, new element #4=w293, index (row) #4=w313, index (col) #4=w309, new element #5=w286, index (row) #5=w313, index (col) #5=w285) -> (w314:string[][])
        n132 = Bundle By Name(cluster=w326, "Dryer Out.Cycle Count"=w323, "Dryer Out.Dryer Details.Cycle Count"=w308, "Dryer Out.Dryer Details.Status"=w322, "Dryer Out.Dryer Details.Debug ASCII"=w321, "Dryer Out.Dryer Details.Total Time On"=w307, "Dryer Out.Hist Record(Cycle Count, t-comp)"=w314) -> (w325:T7)
        n133 = call <vilib>:"Add State(s) to Queue__jki_lib_state_machine.vi"("State(s) in (\"\")"=w329) -> ("States Out"=w328:string)  [unwired: 14 in]
      }
      frame #16 {
        w330 = 1  # Cycle Count (col)
        # "Adds one to count in the sample record, and calls update history data (which creates a new history record)."
        n134 = Unbundle By Name(w337) -> ("Dryer Out.Sample Record(t, CC, ASCII, Status )"=w338:string[], "Dryer Out.Cycle Count"=w335:i32)
        n135 = Increment(x=w335) -> (x+1=w334:i32)
        n136 = Number To Decimal String(number=w334) -> (decimal integer string=w332:string)  [unwired: 1 in]
        n137 = Replace Array Subset(array=w338, new element=w332, index=w330) -> (w333:string[])
        n138 = Bundle By Name(cluster=w337, "Dryer Out.Sample Record(t, CC, ASCII, Status )"=w333, "Dryer Out.Cycle Count"=w334) -> (w336:T7)
        n139 = call <vilib>:"Add State(s) to Queue__jki_lib_state_machine.vi"("State(s) in Front (\"\")"="Update History Data" ("State(s) in Front (\"\")"), "State(s) in (\"\")"=w341) -> ("States Out"=w340:string)  [unwired: 13 in]
      }
    }
  }
  n140 = Unbundle By Name(w2) -> ("Restart Ready?"=→"Restart Ready?":bool)
